vi "Tetromino_MoveDown.vi"(2 "Origin":i16) -> (16 "NewOrigin":i16)   [LabVIEW 2018]
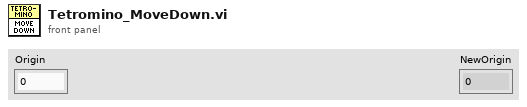
[diagram p1: front panel]
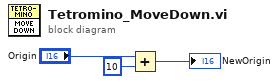
[diagram p0: block diagram]
diagram:
  n1 = Add(x="Origin", y=i16 10) -> (x+y=→"NewOrigin":i16)
